vi "Get BaseType.vi"(8 "error in (no error)":errorcluster, 11 "LVEnum.lvclass in":refnum<class "LVEnum.lvclass">) -> (0 "error out":errorcluster, 2 "BaseType":refnum<class "LVType.lvclass">, 3 "LVEnum.lvclass out":refnum<class "LVEnum.lvclass">)   [LabVIEW 2020, in "LVDataTypes.lvlib" / "LVEnum.lvclass"]
uses:
  <vilib>/AppBuilder/Engine/WebServiceDescription/LVDataTypes/LVEnum/LVEnum.lvclass
  <vilib>/AppBuilder/Engine/WebServiceDescription/LVDataTypes/LVType/LVType.lvclass
  <vilib>/AppBuilder/Engine/WebServiceDescription/LVDataTypes/LVEnum/LVEnum.lvclass/LVEnum.ctl
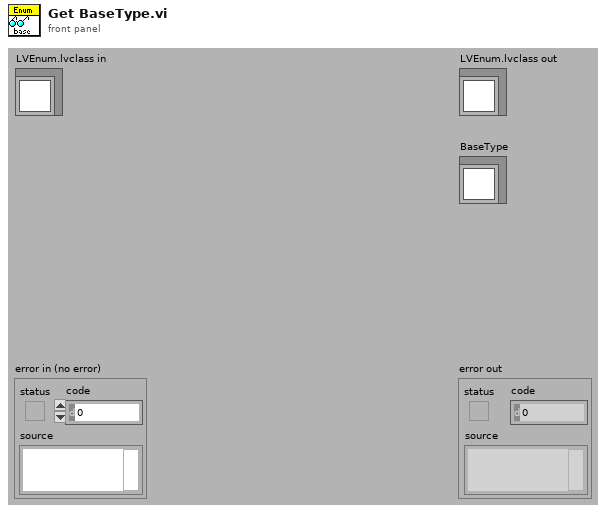
[diagram p1: front panel]
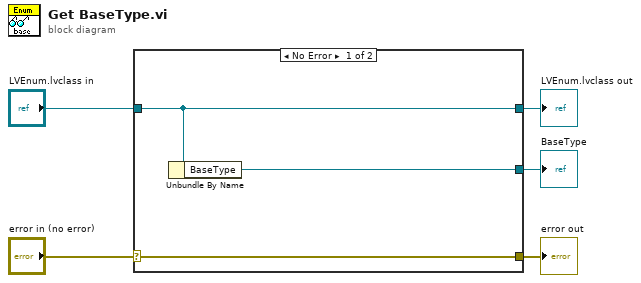
[diagram p0: block diagram]
diagram:
  n1 = case shown="No Error" "error in (no error)" {
    selector: "error in (no error)" -> [w8 w9]
    tunnel: [w8 w9] -> w4
    tunnel: [w7 w10] -> w2
    tunnel: "LVEnum.lvclass in" -> [w7 w10]
    tunnel: [w6 _] -> w1
    frame No Error {
      n2 = Unbundle By Name(w7) -> ("BaseType"=w6:refnum<class "LVType.lvclass">)
    }
    frame Error {
    }
  }
  "error out" <- w4
  "LVEnum.lvclass out" <- w2
  "BaseType" <- w1
